vi "Shut Down.vi"(8 "error in (no error)":errorcluster, 11 "Application in":refnum<class "Application.lvclass">) -> (0 "error out":errorcluster, 3 "Application out":refnum<class "Application.lvclass">)   [LabVIEW 2023, in "Application.lvlib" / "Application.lvclass"]
uses:
  Application.lvclass
  Application.lvclass/Application.ctl
  <vilib>/ActorFramework/Message Enqueuer/Message Enqueuer.lvclass/Message Enqueuer.ctl
  User Interface/Splash Screen Messages/Update Status Msg/Update Status Msg.lvclass/Update Status Msg.ctl
  <vilib>/ActorFramework/Message Enqueuer/Enqueue.vi
  <vilib>/ActorFramework/Stop Msg/Stop Msg.lvclass
  C:/Program Files/National Instruments/LabVIEW 2023/vi.lib/ActorFramework/Message/Message.lvclass
  User Interface/Splash Screen Messages/Update Status Msg/Update Status Msg.lvclass
  <vilib>/ActorFramework/Message Priority Queue/Priority Enqueue.vi
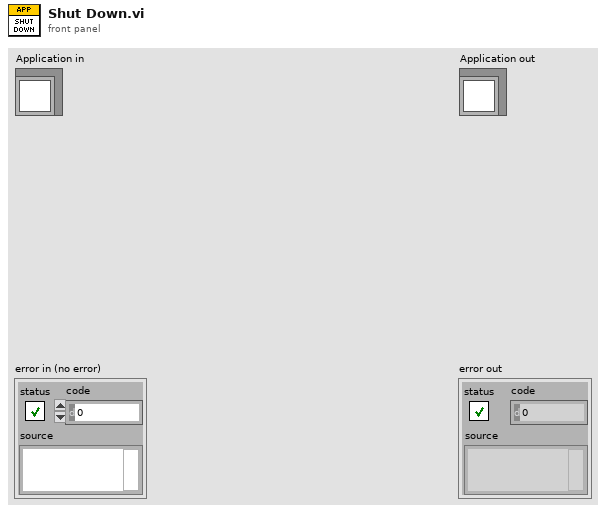
[diagram p1: front panel]
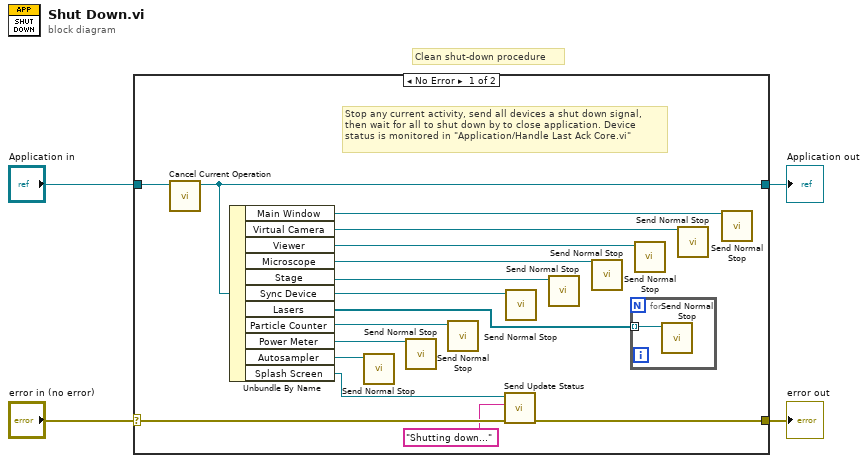
[diagram p0: block diagram]
diagram:
  # "Clean shut-down procedure"
  n1 = case shown="No Error" "error in (no error)" {
    selector: "error in (no error)" -> [w10 w23]
    tunnel: [w9 w23] -> w3
    tunnel: [w19 w22] -> w1
    tunnel: "Application in" -> [w20 w22]
    frame No Error {
      # "Stop any current activity, send all devices a shut down signal,\nthen wait for all to shut down by to close application. Device\nstatus is monitored in \"Application/Handle Last Ack Core.vi\""
      n2 = call-dynamic "Cancel Current Operation.vi"("Application in"=w20) -> ("Application out"=w19:refnum<class "Application.lvclass">)  [unwired: 9 in, 1 out]
      n3 = Unbundle By Name(w19) -> ("Main Window"=w18:refnum<class "Message Enqueuer.lvclass">, "Virtual Camera"=w17:refnum<class "Message Enqueuer.lvclass">, "Viewer"=w16:refnum<class "Message Enqueuer.lvclass">, "Microscope"=w15:refnum<class "Message Enqueuer.lvclass">, "Stage"=w14:refnum<class "Message Enqueuer.lvclass">, "Sync Device"=w13:refnum<class "Message Enqueuer.lvclass">, "Lasers"=w12:refnum<class "Message Enqueuer.lvclass">[], "Particle Counter"=w11:refnum<class "Message Enqueuer.lvclass">, "Power Meter"=w7:refnum<class "Message Enqueuer.lvclass">, "Autosampler"=w5:refnum<class "Message Enqueuer.lvclass">, "Splash Screen"=w6:refnum<class "Message Enqueuer.lvclass">)
      n4 = call <vilib>:"Send Normal Stop.vi"("Message Enqueuer"=w5) -> ()  [unwired: 10 in, 1 out]
      n5 = call <vilib>:"Send Normal Stop.vi"("Message Enqueuer"=w7) -> ()  [unwired: 10 in, 1 out]
      n6 = call <vilib>:"Send Normal Stop.vi"("Message Enqueuer"=w11) -> ()  [unwired: 10 in, 1 out]
      n7 = call "Send Update Status.vi"("error in (no error)"=w10, "Status Message"="Shutting down...", "Message Enqueuer"=w6) -> ("error out"=w9:errorcluster)  [unwired: 7 in, 1 out]
      n8 = call <vilib>:"Send Normal Stop.vi"("Message Enqueuer"=w13) -> ()  [unwired: 10 in, 1 out]
      n9 = call <vilib>:"Send Normal Stop.vi"("Message Enqueuer"=w14) -> ()  [unwired: 10 in, 1 out]
      n10 = call <vilib>:"Send Normal Stop.vi"("Message Enqueuer"=w15) -> ()  [unwired: 10 in, 1 out]
      n11 = for {
        tunnel: w12 -> [w21] mode=indexing
        n12 = call <vilib>:"Send Normal Stop.vi"("Message Enqueuer"=w21) -> ()  [unwired: 10 in, 1 out]
      }
      n13 = call <vilib>:"Send Normal Stop.vi"("Message Enqueuer"=w16) -> ()  [unwired: 10 in, 1 out]
      n14 = call <vilib>:"Send Normal Stop.vi"("Message Enqueuer"=w17) -> ()  [unwired: 10 in, 1 out]
      n15 = call <vilib>:"Send Normal Stop.vi"("Message Enqueuer"=w18) -> ()  [unwired: 10 in, 1 out]
    }
    frame Error {
    }
  }
  "error out" <- w3
  "Application out" <- w1
